vi "B_Init.vi"(8 "error in (no error)":errorcluster, 11 "object in":refnum<class "B.lvclass">) -> (0 "error out":errorcluster, 3 "object out":refnum<class "B.lvclass">)   [LabVIEW 2013, in "B.lvclass"]
uses:
  B.lvclass
  B.lvclass/B.ctl
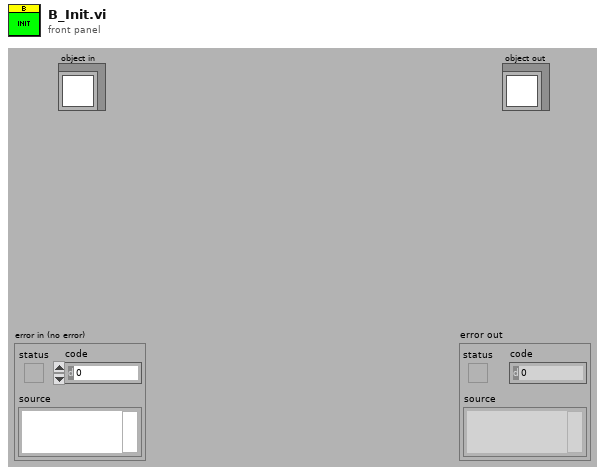
[diagram p1: front panel]
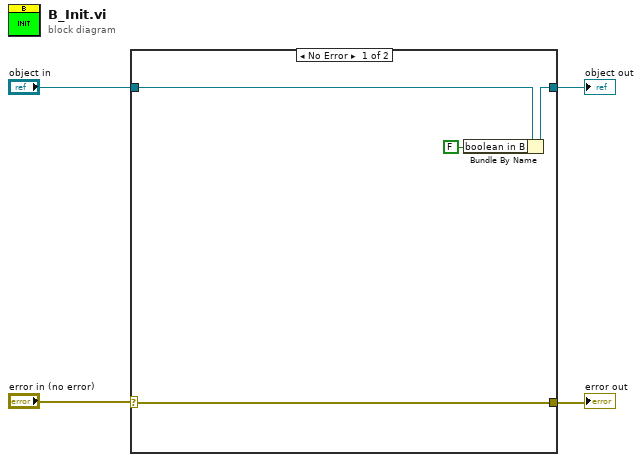
[diagram p0: block diagram]
diagram:
  n1 = case shown="No Error" "error in (no error)" {
    selector: "error in (no error)" -> [w5 w9]
    tunnel: "object in" -> [w8 w10]
    tunnel: [w7 w10] -> w3
    tunnel: [w5 w9] -> w1
    frame No Error {
      n2 = Bundle By Name(cluster=w8, "boolean in B"=FALSE ("None")) -> (w7:refnum<class "B.lvclass">)
    }
    frame Error {
    }
  }
  "object out" <- w3
  "error out" <- w1
